vi "25.04.x-alpha CV Fixer.vi"() -> ()   [LabVIEW 2019]
uses:
  <vilib>/Utility/sysdir.llb/System Directory Type.ctl
  Type defs/Loop data Type Def.ctl
  Type defs/Persistent Type Def.ctl
  Type defs/Temp handle Type Def.ctl
  Type defs/Temp ctrl Type Def.ctl
  Custom devices/Custom temp ctrl settings.ctl
  Type defs/Paths Type Def.ctl
  Type defs/Settings Type Def.ctl
  Type defs/Imps Type Def.ctl
  Type defs/Source-meter Type Def.ctl
  Custom devices/Custom source-meter settings.ctl
  Type defs/Other settings Type Def.ctl
  Type defs/IV properties Type Def.ctl
  Type defs/CV properties Type Def.ctl
  Type defs/DLTS properties Type Def.ctl
  Type defs/LDLTS properties Type Def.ctl
  Type defs/MFIA handle Type Def.ctl
  <instrlib>/Zurich Instruments LabOne/Public/ziTypeHandle.ctl
  <instrlib>/Zurich Instruments LabOne/Public/Modules/ziTypeModHandle.ctl
  Type defs/Source-meter handle Type Def.ctl
  Type defs/Session internal index Type Def.ctl
  Type defs/IV measurement Type Def.ctl
  Type defs/CV measurement Type Def.ctl
  Type defs/LDLTS measurement Type Def.ctl
  Type defs/cDLTS measurement Type Def.ctl
  <instrlib>/Zurich Instruments LabOne/Zurich Instruments LabOne.lvlib
panel:
  out "Progress":i32(slide) scale=0.0..25.0
  in  "File to be fixed":path
  out "Version":dbl caption="Numeric" format="myDLTS %.;%.2g"
  # "This VI can be used to fix the following error in CV data stored in the myDLTS session files:\nIn myDLTS versions 25.04.01-alpha to 25.04.05-alpha CV data is saved multiple times per sweep in blocks.\nMissing (partialy measured) data is padded with NaNs. The actual data is stored in the last block. \nThis VI removes all but the last data block/"
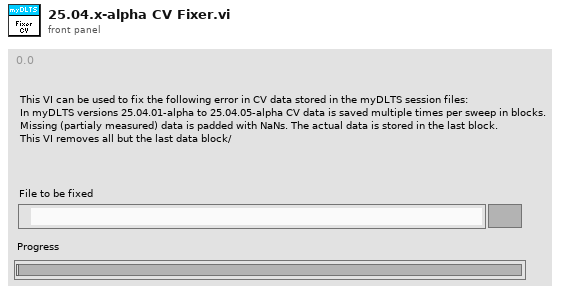
[diagram p1: front panel]
types:
  T1 = typedef "Session internal index Type Def.ctl" = cluster{"IV":T2[], "CV":T4[], "LDLTS":T6[], "Conv DLTS":T8[]}
  T2 = typedef "IV measurement Type Def.ctl" = cluster{"Name":string, "Comment":string, "Time":timestamp, "Folder":path, "IV properties":T3, "GUID":string}
  T3 = typedef "IV properties Type Def.ctl" = cluster{"T":dbl[unit], "Vstart":dbl[unit], "Vstop":dbl[unit], "Vpoints":dbl, "Settling":dbl[unit], "I limit":dbl[unit], "Log mapping":bool, "Averaging":dbl}
  T4 = typedef "CV measurement Type Def.ctl" = cluster{"Name":string, "Comment":string, "Time":timestamp, "Folder":path, "CV properties":T5, "GUID":string}
  T5 = typedef "CV properties Type Def.ctl" = cluster{"T":dbl[unit], "Vstart":dbl[unit], "Vstop":dbl[unit], "Vpoints":dbl, "Precision":enum16{"Low (Fast)", "Normal", "High (Slow)"}, "Test signal":dbl[unit], "Auto I range":bool, "Test frequency":dbl[unit], "I range":dbl, "V range":dbl[unit], "Log mapping":bool, "Rel perm":dbl, "Area":dbl[unit], "Equivalent circuit model":u16}
  T6 = typedef "LDLTS measurement Type Def.ctl" = cluster{"Name":string, "Comment":string, "Time":timestamp, "Folder":path, "LDLTS properties":T7, "GUID":string}
  T7 = typedef "LDLTS properties Type Def.ctl" = cluster{"T":dbl[unit], "Test signal":dbl[unit], "Test frequency":dbl[unit], "Bandwidth":dbl[unit], "Averaging":dbl, "Vbias":dbl[unit], "Vpulse":dbl[unit], "pulse length":dbl[unit], "Pulse 2":bool, "Vpulse 2":dbl[unit], "pulse length 2":dbl[unit], "I range":dbl, "V range":dbl[unit], "Sampling rate":dbl[unit], "Acq. delay":dbl[unit], "Sampling time":dbl[unit], "Filter order":i32, "Equivalent circuit model":u16}
  T8 = typedef "cDLTS measurement Type Def.ctl" = cluster{"Name":string, "Comment":string, "Time":timestamp, "Folder":path, "DLTS properties":T9, "GUID":string}
  T9 = typedef "DLTS properties Type Def.ctl" = cluster{"Tstart":dbl[unit], "Instant start":bool, "Tstop":dbl[unit], "T rate":dbl[unit], "Test signal":dbl[unit], "Test frequency":dbl[unit], "Bandwidth":dbl[unit], "Averaging":dbl, "Vbias":dbl[unit], "Vpulse":dbl[unit], "pulse length":dbl[unit], "Pulse 2":bool, "Vpulse 2":dbl[unit], "pulse length 2":dbl[unit], "I range":dbl, "V range":dbl[unit], "Emission rate":dbl[unit][], "Sampling rate":dbl[unit], "Acq. delay":dbl[unit], "Filter order":i32, "Equivalent circuit model":u16}
  T10 = typedef "Loop data Type Def.ctl" = cluster{"Persistent":T11, "Temp handle":T12, "Paths":T15, "Settings":T16, "Software version":dbl, "MFIA handle":T21, "Source-meter handle":T24}
  T11 = typedef "Persistent Type Def.ctl" = cluster{"Last file":path, "Last user":string, "Users":cluster{"User":string, "Authors directory":path}[]}
  T12 = typedef "Temp handle Type Def.ctl" = cluster{"Connected":bool, "Temp ctrl":T13}
  T13 = typedef "Temp ctrl Type Def.ctl" = cluster{"Gain (P)":dbl, "Reset (I)":dbl, "Rate (D)":dbl, "Stabilization rate":dbl, "Stabilization delta":dbl, "Type":enum16{"Custom", "Lake Shore 325", "Lake Shore 331", "Lake Shore 332", "Lake Shore 335", "Lake Shore 336"}, "Custom temp ctrl":T14, "Lakeshore 325":cluster{"VISA name":refnum<visa-resource-name>, "Loop":u16, "Heater Range":u16, "Heater Resistance":u16, "Sample sensor":u16, "Fast sensor":u16, "Slow sensor":u16}, "Lakeshore 331":cluster{"VISA name":refnum<visa-resource-name>, "Loop":u16, "Heater Range":u16, "Sample sensor":u16, "Fast sensor":u16, "Slow sensor":u16}, "Lakeshore 332":cluster{"VISA name":refnum<visa-resource-name>, "Loop":u16, "Heater Range":u16, "Sample sensor":u16, "Fast sensor":u16, "Slow sensor":u16}, "Lakeshore 335":cluster{"VISA name":refnum<visa-resource-name>, "Loop":u16, "Sample sensor":u16, "Fast sensor":u16, "Slow sensor":u16, "Heater Range":u16, "Output mode":enum16{"Off", "Closed Loop PID", "Zone", "Open Loop", "Monitor Out", "Warmup Supply"}}, "Lakeshore 336":cluster{"VISA name":refnum<visa-resource-name>, "Loop":u16, "Output mode":enum16{"Off", "Closed Loop PID", "Zone", "Open Loop"}, "Max current":dbl, "Heater resistance":u16, "Sample sensor":u16, "Slow sensor":u16, "Fast sensor":u16}}
  T14 = typedef "Custom temp ctrl settings.ctl" = cluster{"VISA resource name":refnum<visa-resource-name>}
  T15 = typedef "Paths Type Def.ctl" = cluster{"Manual":path, "Settings":path, "Persistent":path, "Work dir.":path}
  T16 = typedef "Settings Type Def.ctl" = cluster{"MFIA":T17, "Temp ctrl":T13, "Source-meter":T18, "Other":T20, "Defaults":cluster{"IV properties":T3, "CV properties":T5, "DLTS properties":T9, "LDLTS properties":T7}}
  T17 = typedef "Imps Type Def.ctl" = cluster{"Address":string, "Use compensation":bool, "Shut down gracefully":bool}
  T18 = typedef "Source-meter Type Def.ctl" = cluster{"Type":enum16{"Custom", "Keithley 2600", "Keithley 2400 Series"}, "Custom source-meter":T19, "Keithley 2600":cluster{"VISA name":refnum<visa-resource-name>, "Ignore ID Query":bool, "SMU":enum16{"Channel A", "Channel B"}}, "Keithley 2400 Series":cluster{"VISA name":refnum<visa-resource-name>, "Ignore ID Query":bool}}
  T19 = typedef "Custom source-meter settings.ctl" = cluster{"VISA resource name":refnum<visa-resource-name>}
  T20 = typedef "Other settings Type Def.ctl" = cluster{"Enable OriginLab":bool, "Reader mode":bool, "Auto-save":bool}
  T21 = typedef "MFIA handle Type Def.ctl" = cluster{"ziHandle":T22, "Selected device":string, "ziModHandle":T23}
  T22 = typedef "Zurich Instruments LabOne.lvlib/ziTypeHandle.ctl" = cluster{"handleValid":bool, "Conn":u64, "Path Prefix":string, "Handle":u64, "Connected":bool, "Clockbase(s)":dbl}
  T23 = typedef "Zurich Instruments LabOne.lvlib/ziTypeModHandle.ctl" = cluster{"handleValid":bool, "Conn":u64, "ModHandle":u64, "moduleID":string, "Path Prefix":string}
  T24 = typedef "Source-meter handle Type Def.ctl" = cluster{"Connected":bool, "Source-meter":T18}
  T25 = typedef "System Directory Type.ctl" = i32
  T26 = typedef "Session properties Type Def.ctl" = cluster{"Session name":string, "Comment":string, "User":string, "Software version":dbl, "Created":timestamp, "Modified":timestamp, "Binary":bool, "GUID":string}
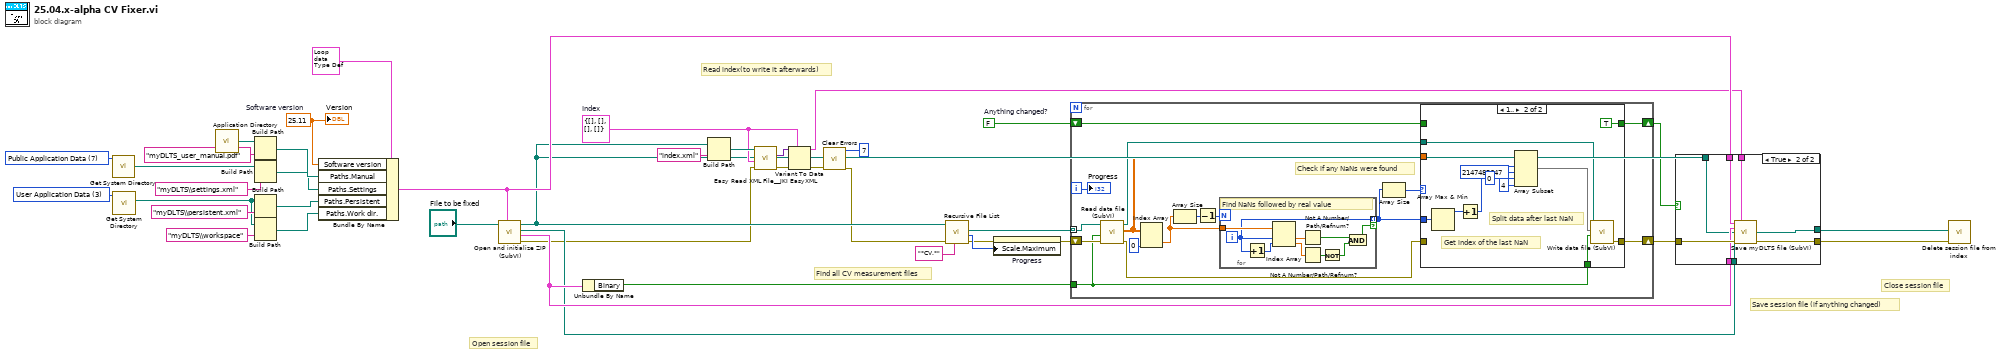
[diagram p0: block diagram]
diagram:
  w2 = FALSE  # Anything changed?
  w13 = T1 {"IV"=[], "CV"=[], "LDLTS"=[], "Conv DLTS"=[]}  # Index
  w27 = 25.11  # Software version
  w29 = T25 7 items=["User Home"=0, "User Desktop"=1, "User Documents"=2, "User Application Data"=3, "User Preferences"=4, "User Temporary"=5, "Public Documents"=6, "Public Application Data"=7, "Public Preferences"=8, "Public Cache"=13, "System Core Libraries"=9, "System Installed Libraries"=10, "Application Files"=11, "Boot Volume Root"=12] ("system directory type")
  w37 = T25 3 items=["User Home"=0, "User Desktop"=1, "User Documents"=2, "User Application Data"=3, "User Preferences"=4, "User Temporary"=5, "Public Documents"=6, "Public Application Data"=7, "Public Preferences"=8, "Public Cache"=13, "System Core Libraries"=9, "System Installed Libraries"=10, "Application Files"=11, "Boot Volume Root"=12] ("system directory type")
  # "Close session file"
  # "Save session file (if anything changed)"
  # "Find all CV measurement files"
  # "Read index(to write it afterwards)"
  # "Open session file"
  n1 = call <vilib>:"Get System Directory.vi"("system directory type"=w29) -> ("system directory"=w28:path)  [unwired: 10 in]
  n2 = call <vilib>:"Get System Directory.vi"("system directory type"=w37) -> ("system directory"=w34:path)  [unwired: 10 in]
  n3 = call <vilib>:"Application Directory.vi"() -> ("Application Directory"=w40:path)
  n4 = Build Path(base path=w40, name or relative path="myDLTS_user_manual.pdf") -> (appended path=w38:path)
  n5 = Build Path(base path=w28, name or relative path="myDLTS\\settings.xml") -> (appended path=w30:path)
  n6 = Build Path(base path=w34, name or relative path="myDLTS\\persistent.xml") -> (appended path=w31:path)
  n7 = Build Path(base path=w34, name or relative path="myDLTS\\workspace") -> (appended path=w32:path)
  n8 = Bundle By Name(cluster=T10 {"Persistent"={"Last file"=path "", "Last user"="", "Users"=[]}, "Temp handle"={"Connected"=FALSE, "Temp ctrl"={"Gain (P)"=0.0, "Reset (I)"=0.0, "Rate (D)"=0.0, "Stabilization rate"=0.0, "Stabilization delta"=0.0, "Type"=enum."Lake Shore 325", "Custom temp ctrl"={"VISA resource name"=""}, "Lakeshore 325"={"VISA name"="", "Loop"=0, "Heater Range"=1, "Heater Resistance"=0, "Sample sensor"=0, "Fast sensor"=0, "Slow sensor"=0}, "Lakeshore 331"={"VISA name"="", "Loop"=1, "Heater Range"=0, "Sample sensor"=0, "Fast sensor"=0, "Slow sensor"=0}, "Lakeshore 332"={"VISA name"="", "Loop"=1, "Heater Range"=0, "Sample sensor"=0, "Fast sensor"=0, "Slow sensor"=0}, "Lakeshore 335"={"VISA name"="", "Loop"=1, "Sample sensor"=0, "Fast sensor"=0, "Slow sensor"=0, "Heater Range"=0, "Output mode"=enum."Off"}, "Lakeshore 336"={"VISA name"="", "Loop"=1, "Output mode"=enum."Off", "Max current"=1.0, "Heater resistance"=1, "Sample sensor"=1, "Slow sensor"=1, "Fast sensor"=1}}}, "Paths"={"Manual"=path "", "Settings"=path "", "Persistent"=path "", "Work dir."=path ""}, "Settings"={"MFIA"={"Address"="", "Use compensation"=FALSE, "Shut down gracefully"=FALSE}, "Temp ctrl"={"Gain (P)"=0.0, "Reset (I)"=0.0, "Rate (D)"=0.0, "Stabilization rate"=0.1, "Stabilization delta"=0.5, "Type"=enum."Custom", "Custom temp ctrl"={"VISA resource name"=""}, "Lakeshore 325"={"VISA name"="", "Loop"=1, "Heater Range"=1, "Heater Resistance"=1, "Sample sensor"=0, "Fast sensor"=0, "Slow sensor"=0}, "Lakeshore 331"={"VISA name"="", "Loop"=1, "Heater Range"=0, "Sample sensor"=0, "Fast sensor"=0, "Slow sensor"=0}, "Lakeshore 332"={"VISA name"="", "Loop"=1, "Heater Range"=0, "Sample sensor"=0, "Fast sensor"=0, "Slow sensor"=0}, "Lakeshore 335"={"VISA name"="", "Loop"=1, "Sample sensor"=0, "Fast sensor"=0, "Slow sensor"=0, "Heater Range"=0, "Output mode"=enum."Off"}, "Lakeshore 336"={"VISA name"="", "Loop"=1, "Output mode"=enum."Off", "Max current"=1.0, "Heater resistance"=1, "Sample sensor"=1, "Slow sensor"=1, "Fast sensor"=1}}, "Source-meter"={"Type"=enum."Custom", "Custom source-meter"={"VISA resource name"=""}, "Keithley 2600"={"VISA name"="", "Ignore ID Query"=FALSE, "SMU"=enum."Channel A"}, "Keithley 2400 Series"={"VISA name"="", "Ignore ID Query"=FALSE}}, "Other"={"Enable OriginLab"=FALSE, "Reader mode"=FALSE, "Auto-save"=FALSE}, "Defaults"={"IV properties"={"T"=300.0, "Vstart"=-3.0, "Vstop"=3.0, "Vpoints"=101.0, "Settling"=0.0, "I limit"=0.001, "Log mapping"=FALSE, "Averaging"=10.0}, "CV properties"={"T"=300.0, "Vstart"=-10.0, "Vstop"=0.0, "Vpoints"=101.0, "Precision"=enum."Normal", "Test signal"=0.1, "Auto I range"=TRUE, "Test frequency"=1000000.0, "I range"=-2.0, "V range"=10.0, "Log mapping"=FALSE, "Rel perm"=0.0, "Area"=0.0, "Equivalent circuit model"=0}, "DLTS properties"={"Tstart"=200.0, "Instant start"=FALSE, "Tstop"=300.0, "T rate"=0.016666666666666666, "Test signal"=0.1, "Test frequency"=1000000.0, "Bandwidth"=50000.0, "Averaging"=10.0, "Vbias"=-4.0, "Vpulse"=0.0, "pulse length"=0.001, "Pulse 2"=FALSE, "Vpulse 2"=0.0, "pulse length 2"=0.001, "I range"=-2.0, "V range"=10.0, "Emission rate"=[10.0, 20.0, 50.0, 100.0, 200.0, 500.0, 1000.0], "Sampling rate"=107142.859375, "Acq. delay"=0.0, "Filter order"=8, "Equivalent circuit model"=0}, "LDLTS properties"={"T"=300.0, "Test signal"=0.1, "Test frequency"=1000000.0, "Bandwidth"=50000.0, "Averaging"=100.0, "Vbias"=-4.0, "Vpulse"=0.0, "pulse length"=0.001, "Pulse 2"=FALSE, "Vpulse 2"=0.0, "pulse length 2"=0.001, "I range"=-2.0, "V range"=10.0, "Sampling rate"=107142.859375, "Acq. delay"=0.0, "Sampling time"=1.25, "Filter order"=8, "Equivalent circuit model"=0}}}, "Software version"=0.0, "MFIA handle"={"ziHandle"={"handleValid"=FALSE, "Conn"=0, "Path Prefix"="", "Handle"=0, "Connected"=FALSE, "Clockbase(s)"=0.0}, "Selected device"="", "ziModHandle"={"handleValid"=FALSE, "Conn"=0, "ModHandle"=0, "moduleID"="", "Path Prefix"=""}}, "Source-meter handle"={"Connected"=FALSE, "Source-meter"={"Type"=enum."Keithley 2600", "Custom source-meter"={"VISA resource name"=""}, "Keithley 2600"={"VISA name"="", "Ignore ID Query"=FALSE, "SMU"=enum."Channel A"}, "Keithley 2400 Series"={"VISA name"="", "Ignore ID Query"=FALSE}}}}, "Software version"=w27, "Paths.Manual"=w38, "Paths.Settings"=w30, "Paths.Persistent"=w31, "Paths.Work dir."=w32) -> (w19:T10)
  n9 = call "Open and initialize ZIP (SubVI).vi"("Loop Data"=w19, "File to be opened"="File to be fixed") -> ("error out"=w8:errorcluster, "Session properties out"=w18:T26, "Opened file"=w17:path, "Workspace target"=w9:path)  [unwired: 6 in]
  n10 = Unbundle By Name(w18) -> ("Binary"=w23:bool)
  n11 = Build Path(base path=w9, name or relative path="index.xml") -> (appended path=w15:path)
  n12 = call <vilib>:"Easy Read XML File__JKI EasyXML.vi"("error in (no error)"=w8, "LabVIEW Data (Type)"=w13, "XML File Path"=w15) -> ("error out"=w11:errorcluster, "LabVIEW Data"=w16:variant)  [unwired: 6 in, 1 out]
  n13 = Variant To Data(error in=w11, type=w13, Variant=w16) -> (data=w6:T1, error out=w10:errorcluster)
  n14 = call <vilib>:"Clear Errors.vi"("error in (no error)"=w10, "specific error code to clear (0: all)"=7) -> ("error out"=w7:errorcluster)  [unwired: 4 in, 1 out]
  n15 = call <vilib>:"Recursive File List.vi"("pattern"="*CV.*", "error in (no error)"=w7, "Folder Path"=w9) -> ("error out"=w4:errorcluster, "Number of Files"=w5:i32, "All Files in Dir"=w24:path[])  [unwired: 4 in, 2 out]
  n16 = property on="Progress" class="Slide (strict)"(error in=w4, "Scale.Maximum"=w5) -> (error out=w3:errorcluster)  [unwired: 1 in, 1 out]
  n17 = for {
    tunnel: w24 -> [w57] mode=indexing
    tunnel: w23 -> [w53]
    shift-right: [w51] -> w22
    shift-left: w3 -> [w56]
    shift-right: [w48] -> w1
    shift-left: w2 -> [w49]
    i -> [w54]
    # "Check if any NaNs were found"
    n18 = call "Read data file (SubVI).vi"("error in"=w56, "Binary"=w53, "file path in"=w57) -> ("error out"=w50:errorcluster, "2D data"=w44:dbl[][], "file path out"=w52:path)  [unwired: 6 in]
    n19 = Index Array(array=w44, index (col)=0 ("index")) -> (element=w42:dbl[])  [unwired: 1 in]
    n20 = Array Size(array=w42) -> (size(s)=w46:i32)
    n21 = Decrement(x=w46) -> (x-1=w47:i32)
    n22 = for {
      N: w47 -> [_]
      tunnel: w42 -> [w66]
      tunnel: [w64] -> w45 mode=indexing if=w58
      i -> [w64]
      # "Find NaNs followed by real value"
      n23 = Increment(x=w64) -> (x+1=w65:i32)
      n24 = Index Array(array=w66, index #1=w64, index #2=w65) -> (element #1=w63:dbl, element #2=w62:dbl)
      n25 = Not A Number/Path/Refnum?(number/path/refnum=w63) -> (NaN/Path/Refnum?=w60:bool)
      n26 = Not A Number/Path/Refnum?(number/path/refnum=w62) -> (NaN/Path/Refnum?=w61:bool)
      n27 = Not(x=w61) -> (.not. x?=w59:bool)
      n28 = And(x=w60, y=w59) -> (x .and. y?=w58:bool)
    }
    n29 = Array Size(array=w45) -> (size(s)=w55:i32)
    n30 = case shown="1.." w55 {
      tunnel: w45 -> [_ w80]
      tunnel: w44 -> [_ w79]
      tunnel: w53 -> [_ w73]
      tunnel: w52 -> [_ w71]
      tunnel: [w68 w70] -> w51
      tunnel: w50 -> [w68 _]
      tunnel: w49 -> [w67 _]
      tunnel: [w67 TRUE ("Anything changed?")] -> w48
      frame 0, Default {
      }
      frame 1.. {
        # "Split data after last NaN"
        # "Get index of the last NaN"
        n31 = Array Max & Min(array=w80) -> (max value=w75:i32)  [unwired: 3 out]
        n32 = Increment(x=w75) -> (x+1=w74:i32)
        n33 = Array Subset(array=w79, index (row)=w74, length (row)=2147483647 ("length"), index (col)=0 ("index"), length (col)=4 ("length")) -> (w72:dbl[][])
        n34 = call "Write data file (SubVI).vi"("Binary"=w73, "2D data"=w72, "file path in"=w71) -> ("error out"=w70:errorcluster)  [unwired: 7 in, 1 out]
      }
    }
    "Progress" <- w54
  }
  n35 = case shown="True" w1 {
    tunnel: w22 -> [w82 w90]
    tunnel: [w82 w89] -> w21
    tunnel: [w81 w88] -> w20
    tunnel: w19 -> [_ w87]
    tunnel: w18 -> [_ w86]
    tunnel: w17 -> [_ w85]
    tunnel: w9 -> [w81 w84]
    tunnel: w6 -> [_ w83]
    frame False {
    }
    frame True {
      n36 = call "Save myDLTS file (SubVI).vi"("Loop data in"=w87, "Index"=w83, "Session properties"=w86, "Workspace path"=w84, "File"=w85, "Error In"=w90) -> ("Workspace out"=w88:path, "Error  out"=w89:errorcluster)  [unwired: 5 in, 3 out]
    }
  }
  n37 = call "Delete session file from index.vi"("Workspace path"=w20, "error in (no error)"=w21) -> ()  [unwired: 7 in, 2 out]
  "Version" <- w27
